vi "Hat Switch Interpreter.vi"(5 "POVs":i16[](array[numeric])) -> (0 "Buttons":bool[](array[boolean]), 1 "Buttons Pressed":bool[](array[boolean]), 2 "Enum Status":T2(ring), 3 "Numeric Status":u8, 4 "Hat Switch Cluster":T1)   [LabVIEW 2014]
panel:
  # "ENUM LAYOUT"
  # "NUMERIC LAYOUT"
  # "North"
  # "1"
  # "Northeast"
  # "2"
  # "Northwest"
  # "8"
  # "West"
  # "East"
  # "7"
  # "3"
  # "Null"
  # "0"
  # "Southwest"
  # "Southeast"
  # "6"
  # "4"
  # "5"
  # "South"
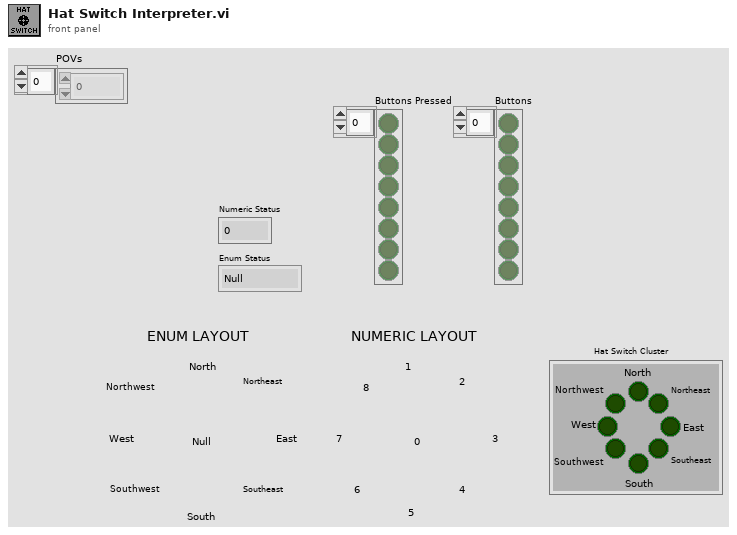
[diagram p1: front panel]
types:
  T1 = cluster{"North":bool, "Northeast":bool, "East":bool, "Southeast":bool, "South":bool, "Southwest":bool, "West":bool, "Northwest":bool}
  T2 = enum8{"Null", "North", "Northeast", "East", "Southeast", "South", "Southwest", "West", "Northwest"}
  T3 = cluster{"North":bool, "Northeast":bool, "East":bool, "Southeast":bool, "South":bool, "Northwest":bool, "Southwest":bool, "West":bool}
  T4 = cluster{"[0]":bool, "[1]":bool, "[2]":bool, "[3]":bool, "[4]":bool, "[5]":bool, "[6]":bool, "[7]":bool, "[8]":bool}
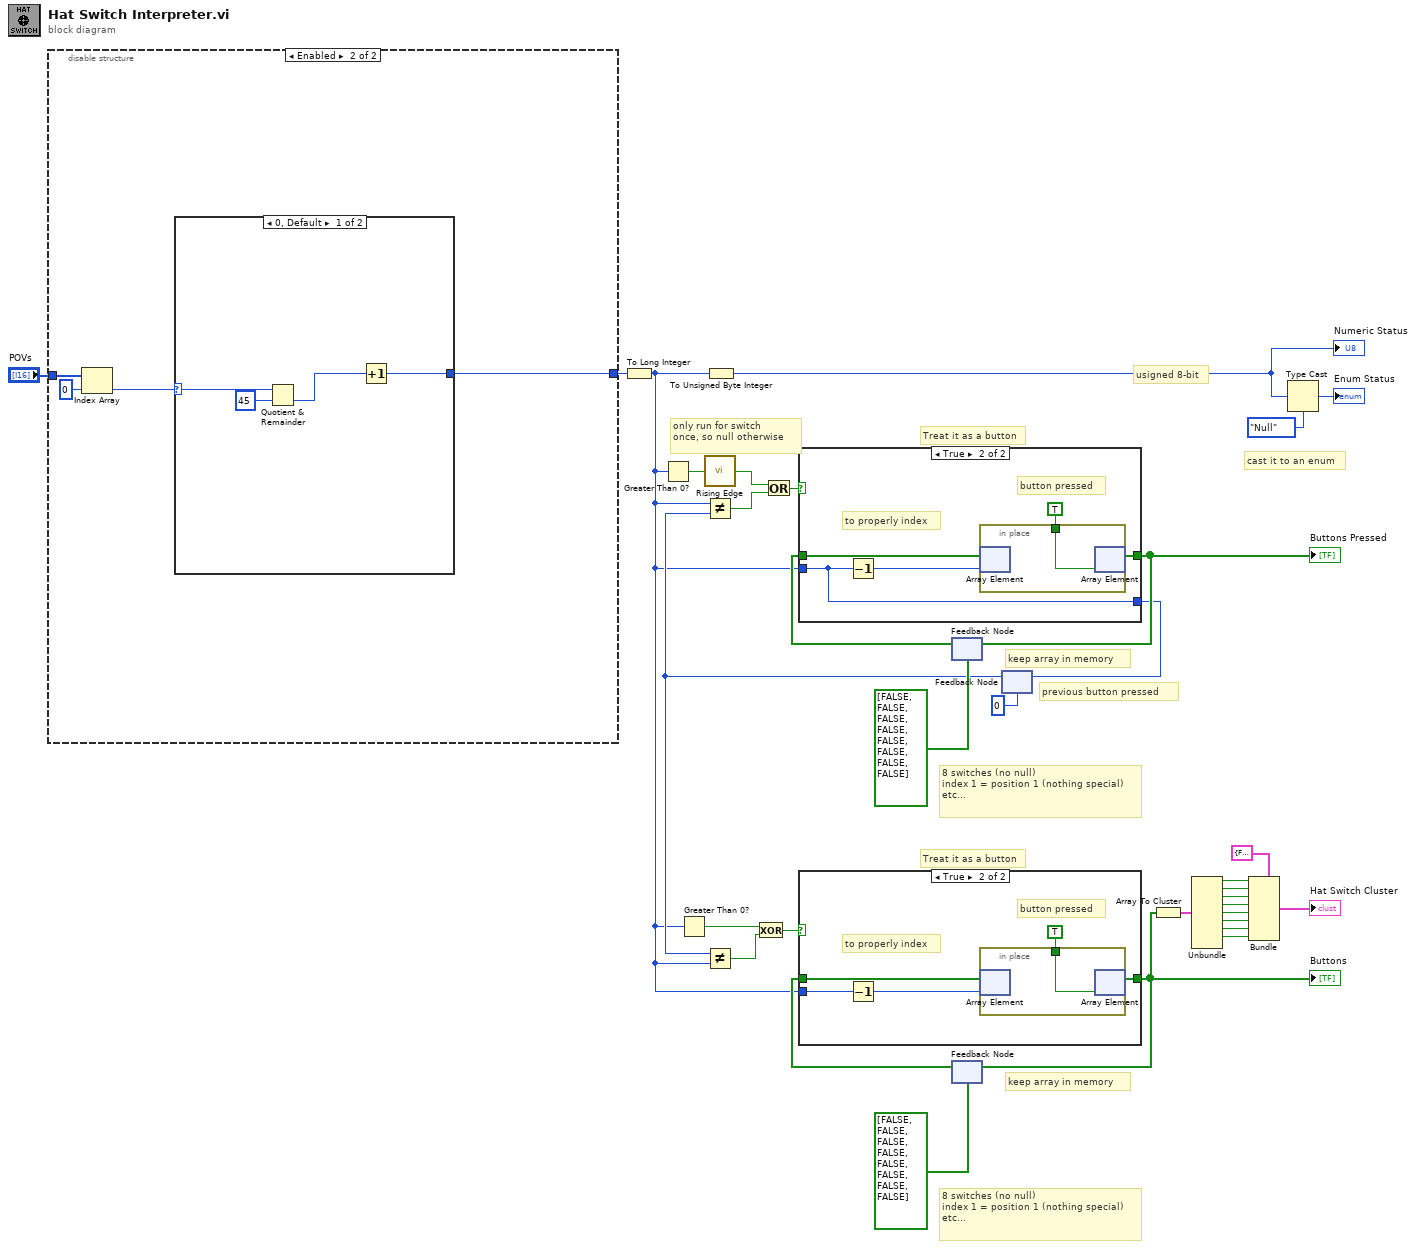
[diagram p0: block diagram]
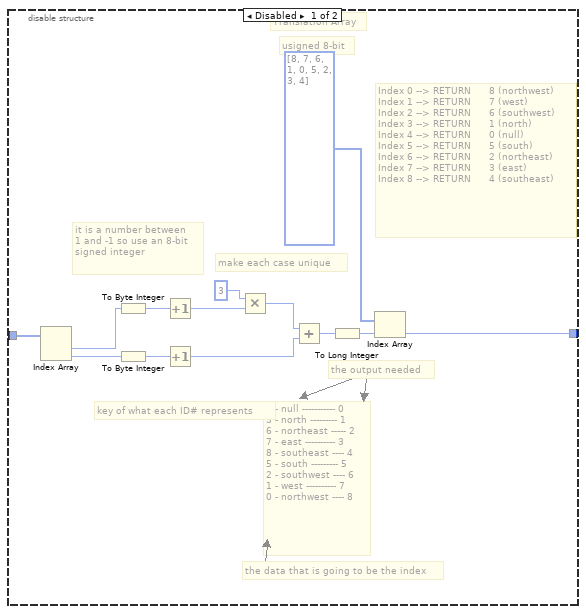
[diagram p2: hidden frame]
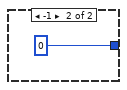
[diagram p3: hidden frame]
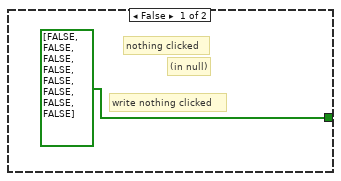
[diagram p4: hidden frame]
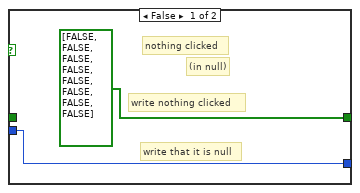
[diagram p5: hidden frame]
diagram:
  # "cast it to an enum"
  # "keep array in memory"
  # "8 switches (no null)\nindex 1 = position 1 (nothing special)\netc..."
  # "Treat it as a button"
  # "only run for switch\nonce, so null otherwise"
  # "keep array in memory"
  # "previous button pressed"
  # "8 switches (no null)\nindex 1 = position 1 (nothing special)\netc..."
  # "Treat it as a button"
  # "usigned 8-bit"
  n1 = disable-structure shown="Enabled" {
    disable-tunnel: [w37 w47] -> w25
    disable-tunnel: "POVs" -> [w36 w50]
    frame Disabled {
      # "usigned 8-bit"
      # "the data that is going to be the index"
      # "the output needed"
      # "key of what each ID# represents"
      # "Index 0 --> RETURN      8 (northwest)\nIndex 1 --> RETURN      7 (west)\nIndex 2 --> RETURN      6 (southwest)\nIndex 3 --> RETURN      1 (north)\nIndex 4 --> RETURN      0 (null)\nIndex 5 --> RETURN      5 (south)\nIndex 6 --> RETURN      2 (northeast)\nIndex 7 --> RETURN      3 (east)\nIndex 8 --> RETURN      4 (southeast)"
      # "4 - null ----------- 0\n3 - north --------- 1\n6 - northeast ----- 2\n7 - east ---------- 3\n8 - southeast ---- 4\n5 - south --------- 5\n2 - southwest ---- 6\n1 - west ---------- 7\n0 - northwest ---- 8"
      # "Translation Array"
      # "it is a number between\n1 and -1 so use an 8-bit\nsigned integer"
      # "make each case unique"
      n2 = Index Array(array=w36) -> (element #1=w35:i16, element #2=w34:i16)  [unwired: 2 in]
      n3 = To Byte Integer(number=w35) -> (8bit integer=w42:i8)
      n4 = To Byte Integer(number=w34) -> (8bit integer=w41:i8)
      n5 = Increment(x=w42) -> (x+1=w46:i8)
      n6 = Increment(x=w41) -> (x+1=w43:i8)
      n7 = Multiply(x=i8 3, y=w46) -> (x*y=w44:i8)
      n8 = Add(x=w44, y=w43) -> (x+y=w39:i8)
      n9 = To Long Integer(number=w39) -> (32bit integer=w38:i32)
      n10 = Index Array(array=u8[] [8, 7, 6, 1, 0, 5, 2, 3, 4], index=w38) -> (element=w37:u8)
    }
    frame Enabled {
      n11 = Index Array(array=w50, index=0) -> (element=w48:i16)
      n12 = case shown="0, Default" w48 {
        selector: w48 -> [w54 _]
        tunnel: [w51 i16 0] -> w47
        frame 0, Default {
          n13 = Quotient & Remainder(x=w54, y=i16 45) -> (floor(x/y)=w52:i16)  [unwired: 1 out]
          n14 = Increment(x=w52) -> (x+1=w51:i16)
        }
        frame -1 {
        }
      }
    }
  }
  n15 = To Long Integer(number=w25) -> (32bit integer=w19:i32)
  n16 = Greater Than 0?(x=w19) -> (x > 0?=w28:bool)
  n17 = Greater Than 0?(x=w19) -> (x > 0?=w21:bool)
  n18 = call "Rising Edge.vi"("Input"=w28) -> ("Rising Edge"=w27:bool)
  n19 = To Unsigned Byte Integer(number=w19) -> (unsigned 8bit integer=w4:u8)
  "Numeric Status" <- w4
  n20 = feedback #1(bool[] [FALSE, FALSE, FALSE, FALSE, FALSE, FALSE, FALSE, FALSE]) -> (w32:bool[])
  n21 = feedback #2(bool[] [FALSE, FALSE, FALSE, FALSE, FALSE, FALSE, FALSE, FALSE]) -> (w23:bool[])
  n22 = feedback #3(0) -> (w20:i32)
  n23 = Not Equal?(x=w19, y=w20) -> (x != y?=w24:bool)
  n24 = Not Equal?(x=w20, y=w19) -> (x != y?=w17:bool)
  n25 = Exclusive Or(1:w17, 2:w21) -> (0:w18:bool)
  n26 = Or(x=w27, y=w24) -> (x .or. y?=w26:bool)
  n27 = case shown="True" w26 {
    tunnel: w32 -> [_ w62]
    tunnel: [bool[] [FALSE, FALSE, FALSE, FALSE, FALSE, FALSE, FALSE, FALSE] w61] -> w31
    tunnel: w19 -> [w57 w58]
    tunnel: [w57 w58] -> w29
    frame False {
      # "write nothing clicked"
      # "write that it is null"
      # "(in null)"
      # "nothing clicked"
    }
    frame True {
      # "to properly index"
      # "button pressed"
      n28 = Decrement(x=w58) -> (x-1=w59:i32)
      n29 = in-place {
        in-place-border: TRUE -> [w63]
        n30 = in-place-array #4(w62, w59) -> ()  [unwired: 1 out]
        n31 = in-place-array #4(w63) -> (w61:bool[])  [unwired: 1 out]
      }
    }
  }
  "Buttons Pressed" <- w31
  n32 = case shown="True" w18 {
    tunnel: w23 -> [_ w69]
    tunnel: [bool[] [FALSE, FALSE, FALSE, FALSE, FALSE, FALSE, FALSE, FALSE] w68] -> w16
    tunnel: w19 -> [_ w65]
    frame False {
      # "write nothing clicked"
      # "(in null)"
      # "nothing clicked"
    }
    frame True {
      # "to properly index"
      # "button pressed"
      n33 = Decrement(x=w65) -> (x-1=w66:i32)
      n34 = in-place {
        in-place-border: TRUE -> [w70]
        n35 = in-place-array #5(w69, w66) -> ()  [unwired: 1 out]
        n36 = in-place-array #5(w70) -> (w68:bool[])  [unwired: 1 out]
      }
    }
  }
  "Buttons" <- w16
  n37 = feedback-in #1(w31) -> ()
  n38 = feedback-in #2(w16) -> ()
  n39 = feedback-in #3(w29) -> ()
  n40 = Array To Cluster(array=w16) -> (cluster=w15:T4)
  n41 = Unbundle(w15) -> ("[0]"=w13:bool, "[1]"=w5:bool, "[2]"=w6:bool, "[3]"=w7:bool, "[4]"=w8:bool, "[5]"=w9:bool, "[6]"=w10:bool, "[7]"=w11:bool)  [unwired: 1 out]
  n42 = Bundle(cluster=T3 {"North"=FALSE, "Northeast"=FALSE, "East"=FALSE, "Southeast"=FALSE, "South"=FALSE, "Northwest"=FALSE, "Southwest"=FALSE, "West"=FALSE} ("Hat Switch Cluster"), "North"=w13, "Northeast"=w5, "East"=w6, "Southeast"=w7, "South"=w8, "Northwest"=w9, "Southwest"=w10, "West"=w11) -> (→"Hat Switch Cluster":T3)
  n43 = Type Cast(type=T2."Null" ("Enum Status"), x=w4) -> (*(type *) &x=→"Enum Status":T2)
